vi "PlaneFit_FBL.vi"(6 "Planing y/n?":bool, 7 "Reset Clicks":bool, 8 "Y PEN":dbl, 9 "Z":dbl, 10 "Nano Z":dbl, 11 "X":dbl) -> (2 "Plane Height (m)":dbl, 3 "Clicks":i32, 5 "Planing Done?":bool)   [LabVIEW 2019]
uses:
  GlobalClicksHeight_FBL.vi
  <userlib>/HapticSTM/HapticSTM.lvlib
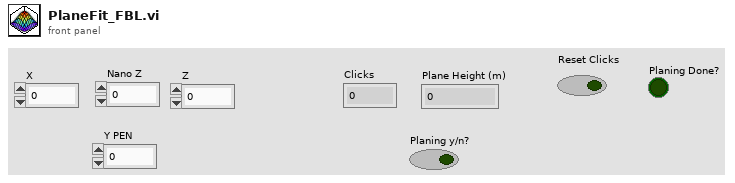
[diagram p1: front panel]
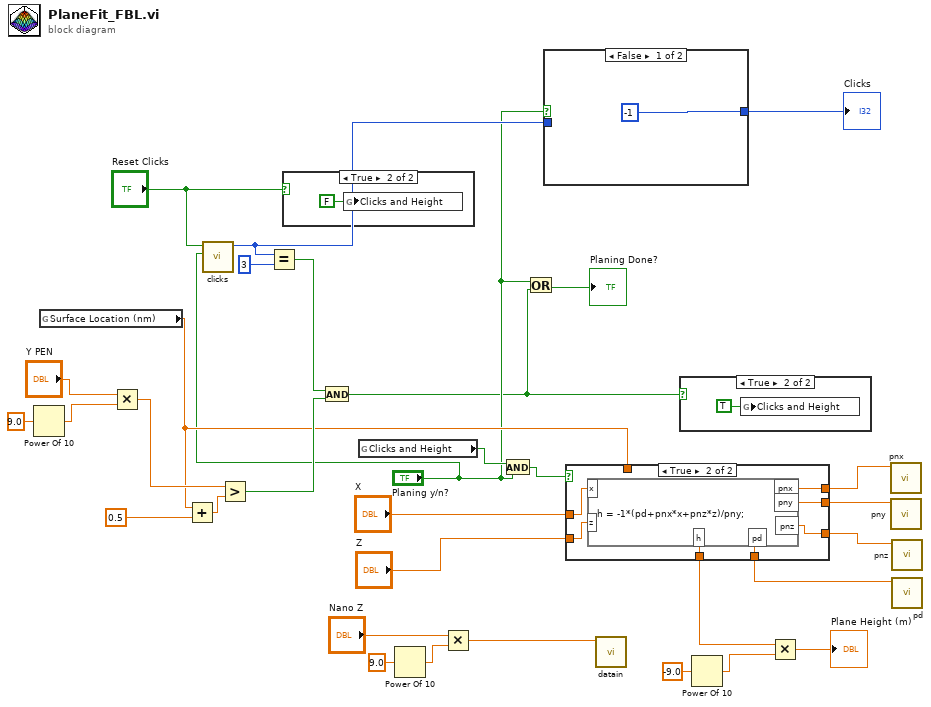
[diagram p0: block diagram]
diagram:
  n1 = Power Of 10(x=9.0) -> (10^x=w20:dbl)
  n2 = global read "GlobalClicksHeight_FBL.vi" "Surface Location (nm)"() -> (w8:dbl)
  n3 = Multiply(x="Y PEN", y=w20) -> (x*y=w17:dbl)
  n4 = Add(x=w8, y=0.5) -> (x+y=w22:dbl)
  n5 = call <userlib>:"clicks.vi"("planing"="Planing y/n?", "reset"="Reset Clicks") -> ("function return"=w5:i32)  [unwired: 9 in]
  n6 = Greater?(x=w17, y=w22) -> (0:w23:bool)
  n7 = Equal?(x=w5, y=3) -> (x = y?=w24:bool)
  n8 = case shown="True" "Reset Clicks" {
    frame False {
    }
    frame True {
      n9 = global write "GlobalClicksHeight_FBL.vi" "Clicks and Height"(FALSE ("Clicks and Height")) -> ()
    }
  }
  n10 = And(x=w24, y=w23) -> (x .and. y?=w1:bool)
  n11 = global read "GlobalClicksHeight_FBL.vi" "Clicks and Height"() -> (w7:bool)
  n12 = Power Of 10(x=9.0) -> (10^x=w16:dbl)
  n13 = Multiply(x="Nano Z", y=w16) -> (x*y=w11:dbl)
  n14 = And(x=w7, y="Planing y/n?") -> (x .and. y?=w6:bool)
  n15 = Or(x="Planing y/n?", y=w1) -> (x .or. y?=→"Planing Done?":bool)
  n16 = case shown="False" "Planing y/n?" {
    tunnel: w5 -> [_ w35]
    tunnel: [-1 ("function return") w35] -> w4
    frame False {
    }
    frame True {
    }
  }
  "Clicks" <- w4
  n17 = call <userlib>:"datain.vi"("output"=w11) -> ()  [unwired: 11 in]
  n18 = case shown="True" w1 {
    frame False {
    }
    frame True {
      n19 = global write "GlobalClicksHeight_FBL.vi" "Clicks and Height"(TRUE ("Clicks and Height")) -> ()
    }
  }
  n20 = Power Of 10(x=-9.0) -> (10^x=w27:dbl)
  n21 = call <userlib>:"pnx.vi"() -> ("function return"=w29:dbl)  [unwired: 11 in]
  n22 = call <userlib>:"pny.vi"() -> ("function return"=w28:dbl)  [unwired: 11 in]
  n23 = call <userlib>:"pnz.vi"() -> ("function return"=w32:dbl)  [unwired: 11 in]
  n24 = call <userlib>:"pd.vi"() -> ("function return"=w31:dbl)  [unwired: 11 in]
  n25 = case shown="True" w6 {
    tunnel: "X" -> [_ w44]
    tunnel: w29 -> [_ w42]
    tunnel: w28 -> [_ w41]
    tunnel: w32 -> [_ w40]
    tunnel: w31 -> [_ w39]
    tunnel: "Z" -> [_ w43]
    tunnel: [w37 w38] -> w12
    tunnel: w8 -> [w37 _]
    frame False {
    }
    frame True {
      n26 = formula code="h = -1*(pd+pnx*x+pnz*z)/pny;"("x"=w44, "z"=w43, "pnx"=w42, "pnz"=w40, "pd"=w39, "pny"=w41) -> ("h"=w38:dbl)
    }
  }
  n27 = Multiply(x=w12, y=w27) -> (x*y=→"Plane Height (m)":dbl)
